vi "5-Mean of an analog signal.vi"() -> ()   [LabVIEW 2019]
uses:
  <vilib>/Analysis/baseanly.llb/Mean (DBL).vi
  <vilib>/Analysis/NI_AALBase.lvlib
panel:
  in  "samples":i32=50
  in  "Time period":u32=500
  out "Mean Value":dbl=-4.5274928806481025 format="%#_3g"
  in  "?":bool
  out "Analog signal":dbl[](graph)=[-43.60028887350222, -61.059295670191574, 33.634455343266964, -90.36869443084497, 38.44535021655242, 67.17207227683937, 69.35937945104807, 1.734160268665974, -5.592899053418277, 78.46611609910634, -55.8819365415567, 8.947054910815533, -15.783356569648443, -68.39805193390855, 91.8406347036042, -86.02515562832558, 29.346073045342447, 0.3809093257320484, 80.03894747928099, -15.078180997625012, 50.207403895308374, -16.454023794491945, -42.9140757814904, -7.272877745200834, 0.4360089420484714, -80.41633143536224, 19.20444529645544, -4.542790164621291, -56.63171876444157, 45.22718381766904, -83.35596025202916, -39.71742129792446, -95.31619945495788, 58.922220030886386, 59.56098943791967, -30.12073541594049, -4.009508435059761, -76.09649408705098, 2.6883545783048746, 13.224566731118736, 42.06739652639884, -24.44266174935312, -12.605303221659625, -42.018720744338765, -79.64776702145949, 86.59622588072165, 0.8120097245567948, 1.416301734960479, 88.69837581049534, -57.45083049510029]
  in  "Amplitude":dbl=100.0 format="%.2p"
  # "MEAN VALUE OF AN ANALOG SIGNAL(NOISE SIGNAL)"
  # "* Samples is the number of samples on waveform\n* Time period is the time after which mean is calculated."
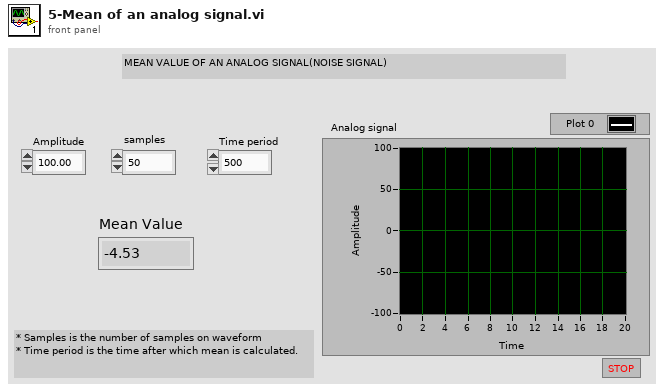
[diagram p1: front panel]
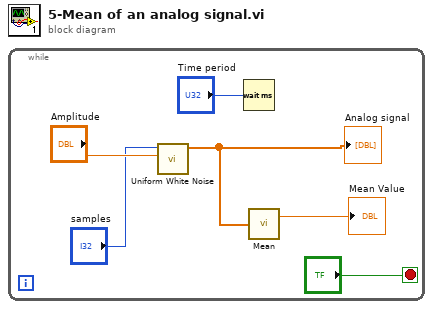
[diagram p0: block diagram]
diagram:
  n1 = while {
    stop <- "?" stop-if-true
    n2 = call <vilib>:"Uniform White Noise.vi"("amplitude"="Amplitude", "samples"="samples") -> ("uniform white noise"=w3:dbl[])  [unwired: 8 in, 1 out]
    "Analog signal" <- w3
    n3 = Wait (ms)(milliseconds to wait="Time period") -> ()  [unwired: 1 out]
    n4 = call-poly <vilib>:"Mean.vi"("X"=w3) -> ("mean"=→"Mean Value":dbl)  [unwired: 1 out]
  }
